vi "get integration time.vi"(8 "error in (no error)":errorcluster, 11 "LineCCD in":refnum<class "LineCCD.lvclass">) -> (0 "error out":errorcluster, 2 "integration time (us)":dbl[unit], 3 "LineCCD out":refnum<class "LineCCD.lvclass">)   [LabVIEW 2012, in "LineCCD.lvclass"]
uses:
  LineCCD.lvclass
  LineCCD.lvclass/LineCCD.ctl
  <instrlib>/ALPHALAS CCD S Series/ALPHALAS CCD S Series.lvlib
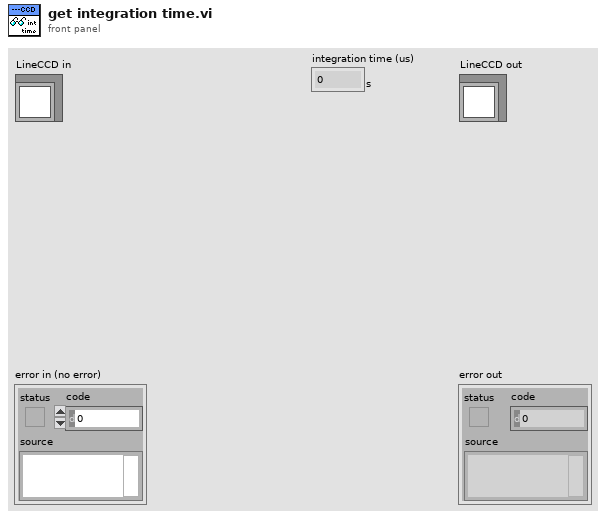
[diagram p1: front panel]
types:
  T1 = typedef "ALPHALAS CCD S Series.lvlib/Integration Time.ctl" = u32
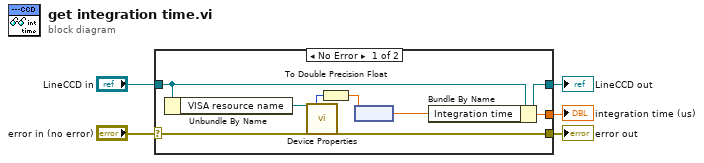
[diagram p0: block diagram]
diagram:
  n1 = case shown="No Error" "error in (no error)" {
    selector: "error in (no error)" -> [w12 w15]
    tunnel: [w11 w15] -> w4
    tunnel: [w9 w14] -> w2
    tunnel: "LineCCD in" -> [w10 w14]
    tunnel: [w6 _] -> w1
    frame No Error {
      n2 = Unbundle By Name(w10) -> ("VISA resource name"=w13:refnum<visa-resource-name>)
      n3 = call <instrlib>:"Device Properties.vi"("VISA resource name"=w13, "error in (no error)"=w12) -> ("Integration Time (µs)"=w8:T1, "error out"=w11:errorcluster)  [unwired: 6 in, 18 out]
      n4 = To Double Precision Float(number=w8) -> (double precision float=w7:dbl)
      n5 = node(w7) -> (w6:dbl[unit])
      n6 = Bundle By Name(cluster=w10, "Integration time"=w6) -> (w9:refnum<class "LineCCD.lvclass">)
    }
    frame Error {
    }
  }
  "error out" <- w4
  "LineCCD out" <- w2
  "integration time (us)" <- w1
